vi "Generate Stop Event.vi"(8 "error in (no error)":errorcluster, 11 "Page":T1=enum."Input Info") -> (0 "error out":errorcluster)   [LabVIEW 2017, in "WebServiceImporter.lvlib" / "Main Panel.lvlib" / "Events.lvlib"]
uses:
  <vilib>/Platform/WebService/Main Panel/Events/Events.lvlib
  <vilib>/Platform/WebService/Main Panel/Events/Data Type/Page.ctl
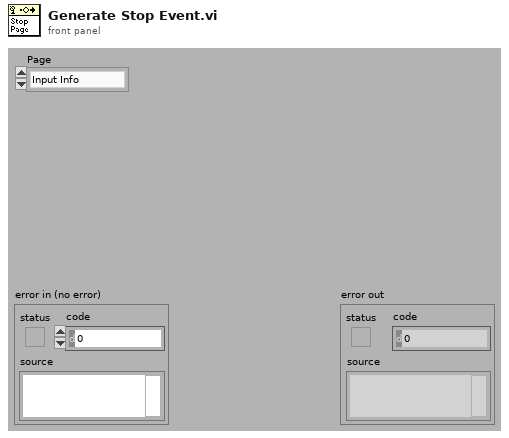
[diagram p1: front panel]
types:
  T1 = typedef "WebServiceImporter.lvlib/Main Panel.lvlib/Events.lvlib/Page.ctl" = enum16{"Input WSDL", "Input Authentication", "Input Info", "Select Methods", "Preview", "Progress", "Finish"}
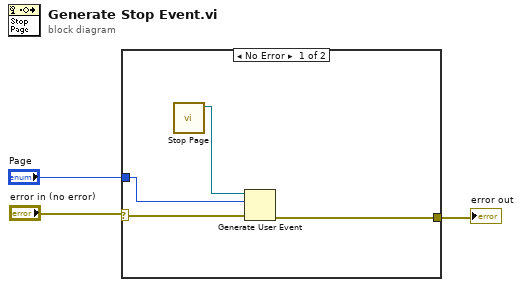
[diagram p0: block diagram]
diagram:
  n1 = case shown="No Error" "error in (no error)" {
    selector: "error in (no error)" -> [w7 w8]
    tunnel: "Page" -> [w5 _]
    tunnel: [w4 w8] -> w1
    frame No Error {
      n2 = call <vilib>:"Stop Page.vi"() -> ("user event (out)"=w6:refnum<user-event>)  [unwired: 11 in]
      n3 = Generate User Event(user event=w6, event data cluster=w5, error in=w7) -> (error out=w4:errorcluster)  [unwired: 1 in, 1 out]
    }
    frame Error {
    }
  }
  "error out" <- w1
